vi "Parser1.vi"(0 "InputString":string="OK arg1 arg2 arg3 arg4") -> (1 "Remainder":string="arg4", 2 "Status":i32, 3 "Arg1 Out":string="arg1", 4 "Arg2 Out":string="arg2", 5 "Arg3 Out":string="arg3", 6 "Arg4 Out":string="arg4")   [LabVIEW 2014]
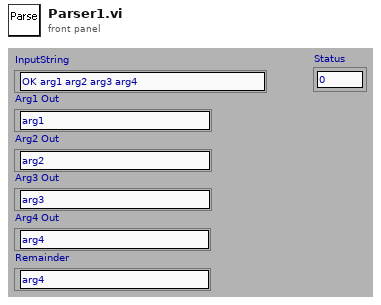
[diagram p1: front panel]
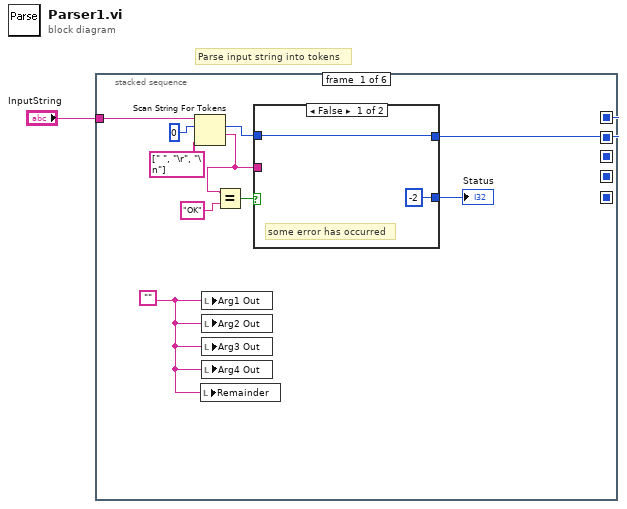
[diagram p0: block diagram]
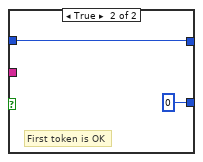
[diagram p2: hidden frame]
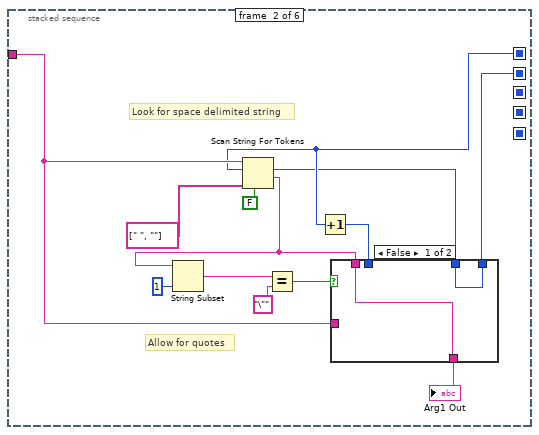
[diagram p3: hidden frame]
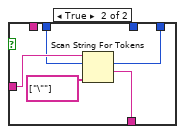
[diagram p4: hidden frame]
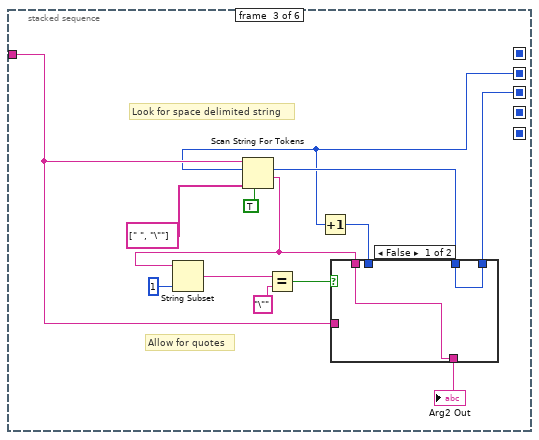
[diagram p5: hidden frame]
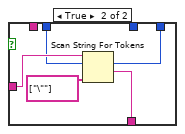
[diagram p6: hidden frame]
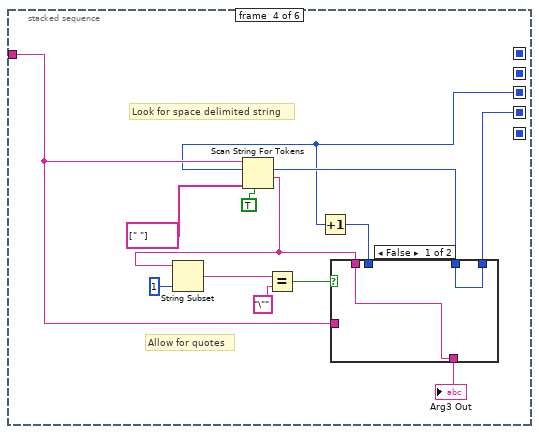
[diagram p7: hidden frame]
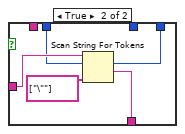
[diagram p8: hidden frame]
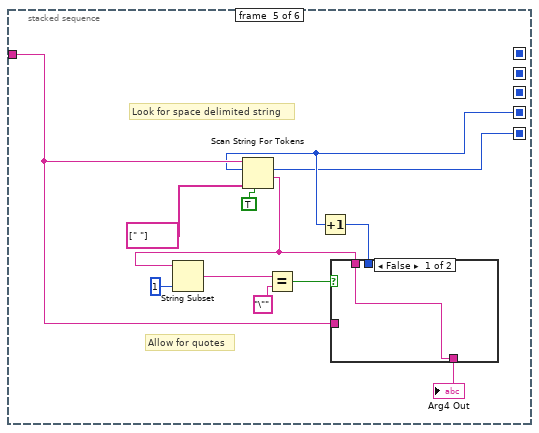
[diagram p9: hidden frame]
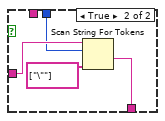
[diagram p10: hidden frame]
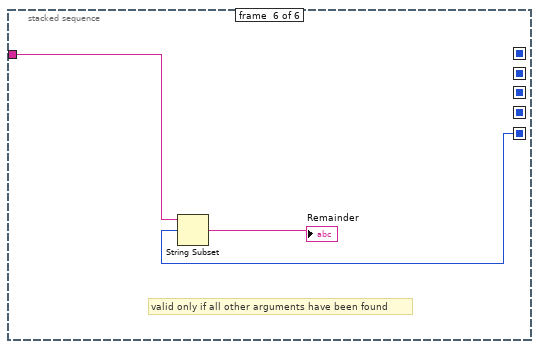
[diagram p11: hidden frame]
diagram:
  # "Parse input string into tokens"
  n1 = stacked-sequence {
    seq-local: [w10 _ _ _ _ _] -> [_ w20 _ _ _ _]
    seq-local: [_ w17 _ _ _ _] -> [_ _ w38 _ _ _]
    seq-local: [_ _ w39 _ _ _] -> [_ _ _ w59 _ _]
    seq-local: [_ _ _ w57 _ _] -> [_ _ _ _ w78 _]
    seq-local: [_ _ _ _ w77 _] -> [_ _ _ _ _ w93]
    tunnel: "InputString" -> [w6 w21 w42 w62 w81 w95]
    frame #0 {
      w2 = ""
      n2 = Scan String For Tokens(6:string[] [" ", "\r", "\n"] ("delimiters (\\s,\\t,\\r,\\n)"), 8:0 ("offset"), 9:w6) -> (1:w3:string, 2:w5:i32)  [unwired: 3 in, 2 out]
      n3 = local write "Remainder"(w2) -> ()
      n4 = local write "Arg1 Out"(w2) -> ()
      n5 = local write "Arg2 Out"(w2) -> ()
      n6 = local write "Arg3 Out"(w2) -> ()
      n7 = local write "Arg4 Out"(w2) -> ()
      n8 = Equal?(x=w3, y="OK") -> (x = y?=w4:bool)
      n9 = case shown="False" w4 {
        tunnel: [w13 w14] -> w10
        tunnel: [-2 0] -> w9
        tunnel: w5 -> [w13 w14]
        tunnel: w3 -> [_ _]
        frame False {
          # "some error has occurred"
        }
        frame True {
          # "First token is OK"
        }
      }
      "Status" <- w9
    }
    frame #1 {
      # "Allow for quotes"
      # "Look for space delimited string"
      n10 = Scan String For Tokens(4:FALSE ("use cached delim/oper data? (F)"), 6:string[] [" ", ""] ("delimiters (\\s,\\t,\\r,\\n)"), 8:w20, 9:w21) -> (1:w22:string, 2:w18:i32)  [unwired: 2 in, 2 out]
      n11 = String Subset(string=w22, length (rest)=1 ("length")) -> (substring=w25:string)  [unwired: 1 in]
      n12 = Equal?(x=w25, y="\"" ("regular expression")) -> (x = y?=w23:bool)
      n13 = Increment(x=w20) -> (x+1=w19:i32)
      n14 = case shown="False" w23 {
        tunnel: [w29 w32] -> w17
        tunnel: [w30 w31] -> w27
        tunnel: w22 -> [w30 _]
        tunnel: w21 -> [_ w35]
        tunnel: w19 -> [_ w34]
        tunnel: w18 -> [w29 _]
        frame False {
        }
        frame True {
          n15 = Scan String For Tokens(6:string[] ["\""] ("delimiters (\\s,\\t,\\r,\\n)"), 8:w34, 9:w35) -> (1:w31:string, 2:w32:i32)  [unwired: 3 in, 2 out]
        }
      }
      "Arg1 Out" <- w27
    }
    frame #2 {
      # "Allow for quotes"
      # "Look for space delimited string"
      n16 = Scan String For Tokens(4:TRUE ("use cached delim/oper data? (F)"), 6:string[] [" ", "\""] ("delimiters (\\s,\\t,\\r,\\n)"), 8:w38, 9:w42) -> (1:w43:string, 2:w40:i32)  [unwired: 2 in, 2 out]
      n17 = String Subset(string=w43, length (rest)=1 ("length")) -> (substring=w46:string)  [unwired: 1 in]
      n18 = Equal?(x=w46, y="\"" ("regular expression")) -> (x = y?=w44:bool)
      n19 = Increment(x=w38) -> (x+1=w41:i32)
      n20 = case shown="False" w44 {
        tunnel: [w49 w52] -> w39
        tunnel: [w50 w51] -> w37
        tunnel: w43 -> [w50 _]
        tunnel: w42 -> [_ w55]
        tunnel: w41 -> [_ w54]
        tunnel: w40 -> [w49 _]
        frame False {
        }
        frame True {
          n21 = Scan String For Tokens(6:string[] ["\""] ("delimiters (\\s,\\t,\\r,\\n)"), 8:w54, 9:w55) -> (1:w51:string, 2:w52:i32)  [unwired: 3 in, 2 out]
        }
      }
      "Arg2 Out" <- w37
    }
    frame #3 {
      # "Allow for quotes"
      # "Look for space delimited string"
      n22 = Scan String For Tokens(4:TRUE ("use cached delim/oper data? (F)"), 6:string[] [" "] ("delimiters (\\s,\\t,\\r,\\n)"), 8:w59, 9:w62) -> (1:w63:string, 2:w60:i32)  [unwired: 2 in, 2 out]
      n23 = String Subset(string=w63, length (rest)=1 ("length")) -> (substring=w66:string)  [unwired: 1 in]
      n24 = Equal?(x=w66, y="\"" ("regular expression")) -> (x = y?=w64:bool)
      n25 = Increment(x=w59) -> (x+1=w61:i32)
      n26 = case shown="False" w64 {
        tunnel: [w69 w72] -> w57
        tunnel: [w70 w71] -> w58
        tunnel: w63 -> [w70 _]
        tunnel: w62 -> [_ w75]
        tunnel: w61 -> [_ w74]
        tunnel: w60 -> [w69 _]
        frame False {
        }
        frame True {
          n27 = Scan String For Tokens(6:string[] ["\""] ("delimiters (\\s,\\t,\\r,\\n)"), 8:w74, 9:w75) -> (1:w71:string, 2:w72:i32)  [unwired: 3 in, 2 out]
        }
      }
      "Arg3 Out" <- w58
    }
    frame #4 {
      # "Allow for quotes"
      # "Look for space delimited string"
      n28 = Scan String For Tokens(4:TRUE ("use cached delim/oper data? (F)"), 6:string[] [" "] ("delimiters (\\s,\\t,\\r,\\n)"), 8:w78, 9:w81) -> (1:w82:string, 2:w77:i32)  [unwired: 2 in, 2 out]
      n29 = String Subset(string=w82, length (rest)=1 ("length")) -> (substring=w85:string)  [unwired: 1 in]
      n30 = Equal?(x=w85, y="\"" ("regular expression")) -> (x = y?=w83:bool)
      n31 = Increment(x=w78) -> (x+1=w80:i32)
      n32 = case shown="False" w83 {
        tunnel: [w88 w89] -> w79
        tunnel: w82 -> [w88 _]
        tunnel: w81 -> [_ w92]
        tunnel: w80 -> [_ w91]
        frame False {
        }
        frame True {
          n33 = Scan String For Tokens(6:string[] ["\""] ("delimiters (\\s,\\t,\\r,\\n)"), 8:w91, 9:w92) -> (1:w89:string)  [unwired: 3 in, 3 out]
        }
      }
      "Arg4 Out" <- w79
    }
    frame #5 {
      # "valid only if all other arguments have been found"
      n34 = String Subset(string=w95, offset (0)=w93) -> (substring=→"Remainder":string)  [unwired: 1 in]
    }
  }
